vi "EventDataToPhotonInfos.vi"(8 "Error In":errorcluster, 10 "Data":u32[](array[numeric])) -> (0 "Error Out":errorcluster, 4 "Photon Infos":T1(array[cluster]))   [LabVIEW 2017]
doc: "This VI analyses a given photon data array for photon information like micro time, macro time, marker information, photon validity, macro time overflow and routing channel number.\n\ninfo@becker-hickl.com"
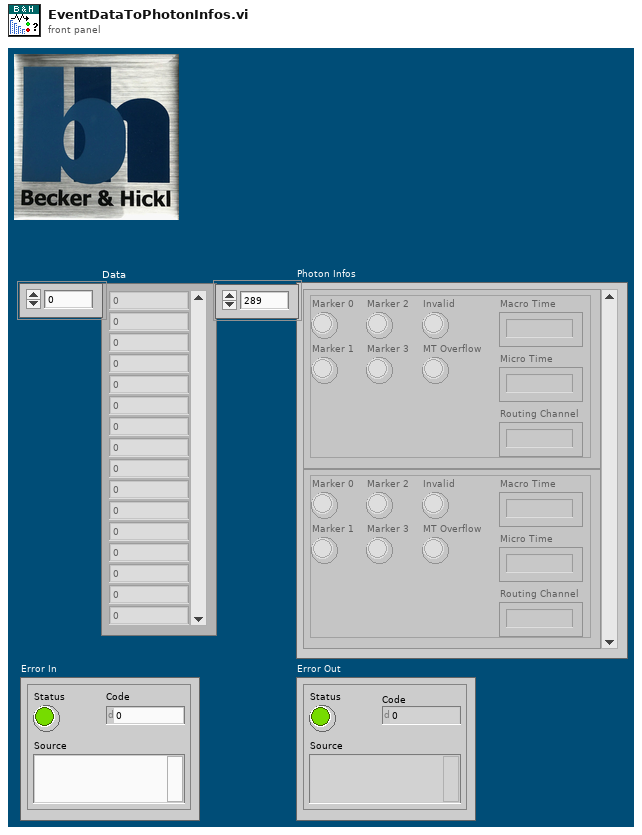
[diagram p1: front panel]
types:
  T1 = cluster{"MT Overflow":bool, "Invalid":bool, "Routing Channel":u32, "Micro Time":u32, "Macro Time":u32, "Marker 3":bool, "Marker 2":bool, "Marker 1":bool, "Marker 0":bool}[]
  T2 = cluster{"MT Overflow":bool, "Invalid":bool, "Routing Channel":u32, "Micro Time":u32, "Macro Time":u32, "Marker 3":bool, "Marker 2":bool, "Marker 1":bool, "Marker 0":bool}
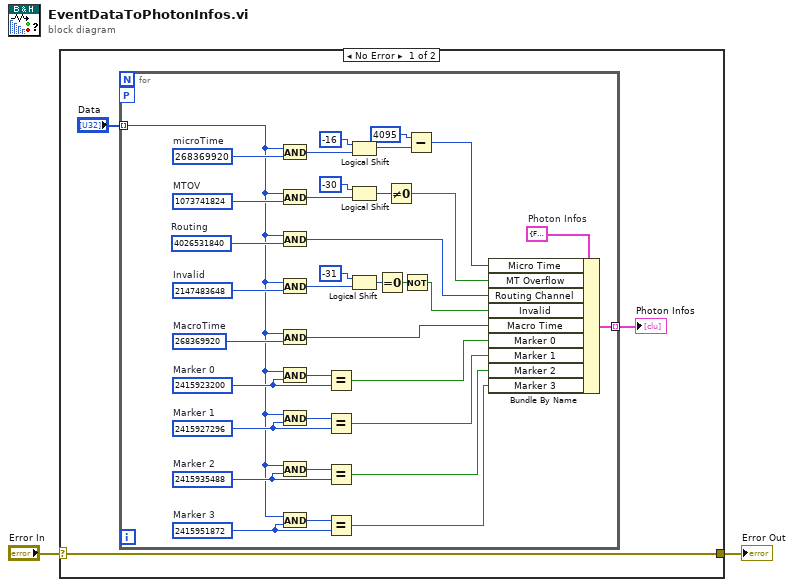
[diagram p0: block diagram]
diagram:
  n1 = case shown="No Error" "Error In" {
    selector: "Error In" -> [w3 w42]
    tunnel: [w3 w42] -> w2
    frame No Error {
      n2 = for {
        tunnel: "Data" -> [w6] mode=indexing
        workers-P: _ -> [_]
        tunnel: [w23] -> w4 mode=indexing
        w9 = u32 2415951872  # Marker 3
        w10 = u32 2415935488  # Marker 2
        w13 = u32 2415927296  # Marker 1
        w17 = u32 2415923200  # Marker 0
        w20 = u32 4026531840  # Routing
        w22 = u32 268369920  # MacroTime
        w28 = T2 {"MT Overflow"=FALSE, "Invalid"=FALSE, "Routing Channel"=0, "Micro Time"=0, "Macro Time"=0, "Marker 3"=FALSE, "Marker 2"=FALSE, "Marker 1"=FALSE, "Marker 0"=FALSE}  # Photon Infos
        w30 = u32 1073741824  # MTOV
        w33 = u32 2147483648  # Invalid
        w37 = u32 268369920  # microTime
        n3 = And(x=w6, y=w37) -> (x .and. y?=w39:u32)
        n4 = And(x=w6, y=w30) -> (x .and. y?=w29:u32)
        n5 = And(x=w6, y=w20) -> (x .and. y?=w19:u32)
        n6 = And(x=w6, y=w33) -> (x .and. y?=w34:u32)
        n7 = And(x=w6, y=w22) -> (x .and. y?=w21:u32)
        n8 = And(x=w6, y=w17) -> (x .and. y?=w18:u32)
        n9 = And(x=w6, y=w13) -> (x .and. y?=w15:u32)
        n10 = And(x=w6, y=w10) -> (x .and. y?=w14:u32)
        n11 = And(x=w6, y=w9) -> (x .and. y?=w8:u32)
        n12 = Equal?(x=w18, y=w17) -> (x = y?=w16:bool)
        n13 = Equal?(x=w15, y=w13) -> (x = y?=w12:bool)
        n14 = Equal?(x=w14, y=w10) -> (x = y?=w11:bool)
        n15 = Equal?(x=w8, y=w9) -> (x = y?=w7:bool)
        n16 = Logical Shift(y=-16, x=w39) -> (x << y=w40:u32)
        n17 = Logical Shift(y=-30, x=w29) -> (x << y=w32:u32)
        n18 = Logical Shift(y=-31, x=w34) -> (x << y=w35:u32)
        n19 = Equal To 0?(x=w35) -> (x = 0?=w26:bool)
        n20 = Not Equal To 0?(x=w32) -> (x != 0?=w27:bool)
        n21 = Not(x=w26) -> (.not. x?=w25:bool)
        n22 = Subtract(x=u32 4095, y=w40) -> (x-y=w24:u32)
        n23 = Bundle By Name(cluster=w28, "Micro Time"=w24, "MT Overflow"=w27, "Routing Channel"=w19, "Invalid"=w25, "Macro Time"=w21, "Marker 0"=w16, "Marker 1"=w12, "Marker 2"=w11, "Marker 3"=w7) -> (w23:T2)
      }
      "Photon Infos" <- w4
    }
    frame Error {
    }
  }
  "Error Out" <- w2
